vi "Pre Launch Init.vi"(11 "Mediator in":refnum<class "Mediator.lvclass">) -> (0 "error out":errorcluster, 3 "Mediator out":refnum<class "Mediator.lvclass">)   [LabVIEW 2020, in "MVA Framework.lvlib" / "Mediator.lvlib" / "Mediator.lvclass"]
doc: "(<B>Filename</B>: Actor Framework.lvlib:Actor.lvclass:Pre Launch Init.vi)\n\nDefines behavior that occurs after the Launch Nested Actor method is invoked but before the actor's Actor Core method begins running.\n\nBy default, this method does nothing. A descendant class may override it to define behavior."
uses:
  Mediator.lvclass
  TopicLookupTable/TopicLookupTable.lvclass
  Mediator.lvclass/Mediator.ctl
  IMediator/IMediator/IMediator.lvclass
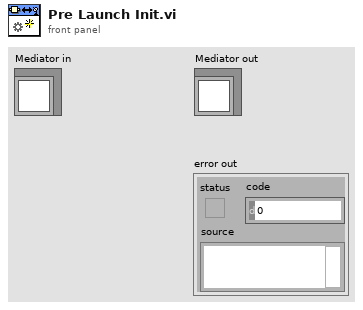
[diagram p1: front panel]
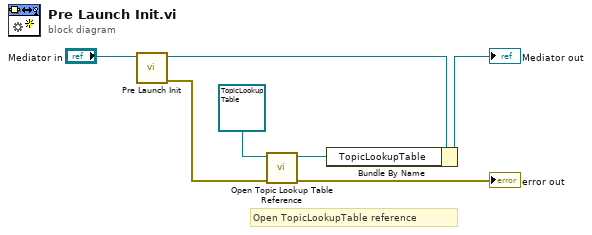
[diagram p0: block diagram]
diagram:
  # "Open TopicLookupTable reference"
  n1 = call-parent "Pre Launch Init.vi"("IMediator In"="Mediator in") -> ("error out"=w4:errorcluster, "IMediator Out"=w7:refnum<class "Mediator.lvclass">)  [unwired: 9 in]
  n2 = call "Open Topic Lookup Table Reference.vi"("error in (no error)"=w4, "TopicLookupTable in"=refnum<class "TopicLookupTable.lvclass"> refnum ("Mediator.lvlib:TopicLookupTable.lvclass")) -> ("error out"=→"error out":errorcluster, "TopicLookupTable Reference"=w5:refnum<data-value>)  [unwired: 8 in]
  n3 = Bundle By Name(cluster=w7, "TopicLookupTable"=w5) -> (→"Mediator out":refnum<class "Mediator.lvclass">)
